vi "Bildaufnahme_Oben.vi"(8 "Fehler in":errorcluster, 11 "Cluster in":T1={"Initialisierung"={"Online?"=FALSE, "Grundpfad"=path "", "Kamera Oben"="", "IP-Adresse Flüssiglinse"="", "Flüssiglinse"=refnum, "Kamera Unten"="", "IP-Adresse SPS"="", "SPS-Verbindung"={"TCP Connection Ref"=refnum, "IP address"="", "timeout ms"=5000, "Connected?"=FALSE, "PLC Type"=enum."S7 1200", "Rack S7 400"=0, "Slot S7 400"=0, "PDU Size"=0, "connection semaphore"=refnum}, "IP-Adresse Lichtgitter"="", "Lichtgitter"=refnum, "Skalierungsfaktor"=0.0, "Bilder Oben"=[], "Bild Unten"=refnum, "Bild Ausschnitt Unten"=refnum}, "Einstellungen"={"Gesamtablauf gestartet"=FALSE, "i. O. Bilder speichern"=FALSE, "Bildspeicherung Offline"=FALSE, "Ausgewähltes Offline-Datum"="", "Ausgewähltes Offline-Teil"="", "Speicherpfad Bilder"=path ""}, "Artikeldaten"={"Artikelnummer"="", "Fertigungsauftrag"="", "Muster ISO"=refnum, "Belichtungszeit Referenzmarken"=0.0, "Fokus Referenzmarken"=0.0, "Belichtungszeit ISO"=0.0, "Fokus ISO"=0.0, "Belichtungszeit Unten"=0.0, "Kontaktanzahl"=0, "Aktueller Kontakt"=0, "Kontaktposition"={"x"=0.0, "y"=0.0}, "Winkel ISO"=0.0, "ISO-Muster nicht vorhanden"=FALSE}, "Werte Kamera Oben"={"Koordinatensystem"={"Punkt x-Achse"={"X"=0.0, "Y"=0.0}, "Ursprung"={"X"=0.0, "Y"=0.0}, "Punkt y-Achse"={"X"=0.0, "Y"=0.0}}, "Position Kontakt"={"x"=0.0, "y"=0.0}, "Winkel Kontakt"=0.0}, "Werte Kamera Unten"={"Prüfung Unten n. i. O."=FALSE}, "Werte Lichtgitter"={"Messwerte Referenzmarken"=[], "Mittelpunkt Referenzmarken"={"x"=0.0, "y"=0.0}, "Messwerte Kontakt"=[], "Offset"={"x"=0.0, "y"=0.0}}, "Rückmeldungen"={"Koordinaten ermittelt"=FALSE, "Vermessung Lichtgitter fertig"=FALSE, "Nachkontrolle Kamera Unten fertig"=FALSE}, "Fehler"={"Referenzen nicht gefunden"=FALSE, "Kontakt nicht gefunden"=FALSE, "Referenzen nicht in Lichtgitter"=FALSE, "Kontakt zu groß"=FALSE, "Kontakt zu klein"=FALSE}, "Statistik"={"Statistiken"=[]}, "Timer"={"Timer Start Position"=0, "Timer Start Lichtgitter"=0, "Timer Start Kamera Unten"=0}}) -> (0 "Fehler out":errorcluster, 3 "Cluster out":T1={"Initialisierung"={"Online?"=FALSE, "Grundpfad"=path "", "Kamera Oben"="", "IP-Adresse Flüssiglinse"="", "Flüssiglinse"=refnum, "Kamera Unten"="", "IP-Adresse SPS"="", "SPS-Verbindung"={"TCP Connection Ref"=refnum, "IP address"="", "timeout ms"=5000, "Connected?"=FALSE, "PLC Type"=enum."S7 1200", "Rack S7 400"=0, "Slot S7 400"=0, "PDU Size"=0, "connection semaphore"=refnum}, "IP-Adresse Lichtgitter"="", "Lichtgitter"=refnum, "Skalierungsfaktor"=0.0, "Bilder Oben"=[], "Bild Unten"=refnum, "Bild Ausschnitt Unten"=refnum}, "Einstellungen"={"Gesamtablauf gestartet"=FALSE, "i. O. Bilder speichern"=FALSE, "Bildspeicherung Offline"=FALSE, "Ausgewähltes Offline-Datum"="", "Ausgewähltes Offline-Teil"="", "Speicherpfad Bilder"=path ""}, "Artikeldaten"={"Artikelnummer"="", "Fertigungsauftrag"="", "Muster ISO"=refnum, "Belichtungszeit Referenzmarken"=0.0, "Fokus Referenzmarken"=0.0, "Belichtungszeit ISO"=0.0, "Fokus ISO"=0.0, "Belichtungszeit Unten"=0.0, "Kontaktanzahl"=0, "Aktueller Kontakt"=0, "Kontaktposition"={"x"=0.0, "y"=0.0}, "Winkel ISO"=0.0, "ISO-Muster nicht vorhanden"=FALSE}, "Werte Kamera Oben"={"Koordinatensystem"={"Punkt x-Achse"={"X"=0.0, "Y"=0.0}, "Ursprung"={"X"=0.0, "Y"=0.0}, "Punkt y-Achse"={"X"=0.0, "Y"=0.0}}, "Position Kontakt"={"x"=0.0, "y"=0.0}, "Winkel Kontakt"=0.0}, "Werte Kamera Unten"={"Prüfung Unten n. i. O."=FALSE}, "Werte Lichtgitter"={"Messwerte Referenzmarken"=[], "Mittelpunkt Referenzmarken"={"x"=0.0, "y"=0.0}, "Messwerte Kontakt"=[], "Offset"={"x"=0.0, "y"=0.0}}, "Rückmeldungen"={"Koordinaten ermittelt"=FALSE, "Vermessung Lichtgitter fertig"=FALSE, "Nachkontrolle Kamera Unten fertig"=FALSE}, "Fehler"={"Referenzen nicht gefunden"=FALSE, "Kontakt nicht gefunden"=FALSE, "Referenzen nicht in Lichtgitter"=FALSE, "Kontakt zu groß"=FALSE, "Kontakt zu klein"=FALSE}, "Statistik"={"Statistiken"=[]}, "Timer"={"Timer Start Position"=0, "Timer Start Lichtgitter"=0, "Timer Start Kamera Unten"=0}})   [LabVIEW 2024]
doc: "Nimmt die Bilder für die Prüfung Oben auf, bzw. lädt die Bilder aus den Dateien wenn im \"Offline-Modus\"."
uses:
  Cluster.ctl
  Kontaktmontagemodul.exe/1abvi3w/vi.lib/userDefined/High Color/IMAQdx.ctl
  Kontaktmontagemodul.exe/1abvi3w/vi.lib/DATA AHEAD/SP7/typedefs/S7 Connection.ctl
  Kontaktmontagemodul.exe/1abvi3w/vi.lib/DATA AHEAD/SP7/typedefs/PLC Type.ctl
  Kontaktmontagemodul.exe/1abvi3w/vi.lib/vision/Image Controls.llb/IMAQ Image.ctl
  Koordinatensystem.ctl
  Statistik.ctl
  Kontaktmontagemodul.exe/1abvi3w/vi.lib/vision/driver/IMAQdx.llb/IMAQdx Buffer Number Mode.ctl
  <resource>/objmgr/imaqdx.rc
  Kontaktmontagemodul.exe/1abvi3w/vi.lib/vision/driver/NI_Vision_Acquisition_Software.lvlib
  Kontaktmontagemodul.exe/1abvi3w/vi.lib/vision/NI_Vision_Development_Module.lvlib
  Kontaktmontagemodul.exe/1abvi3w/vi.lib/DATA AHEAD/SP7/SP7.lvlib
panel:
  in  "Angle":i32
  in  "Angle inkrement":i32
  in  "Zeit für Fokus":u32=300
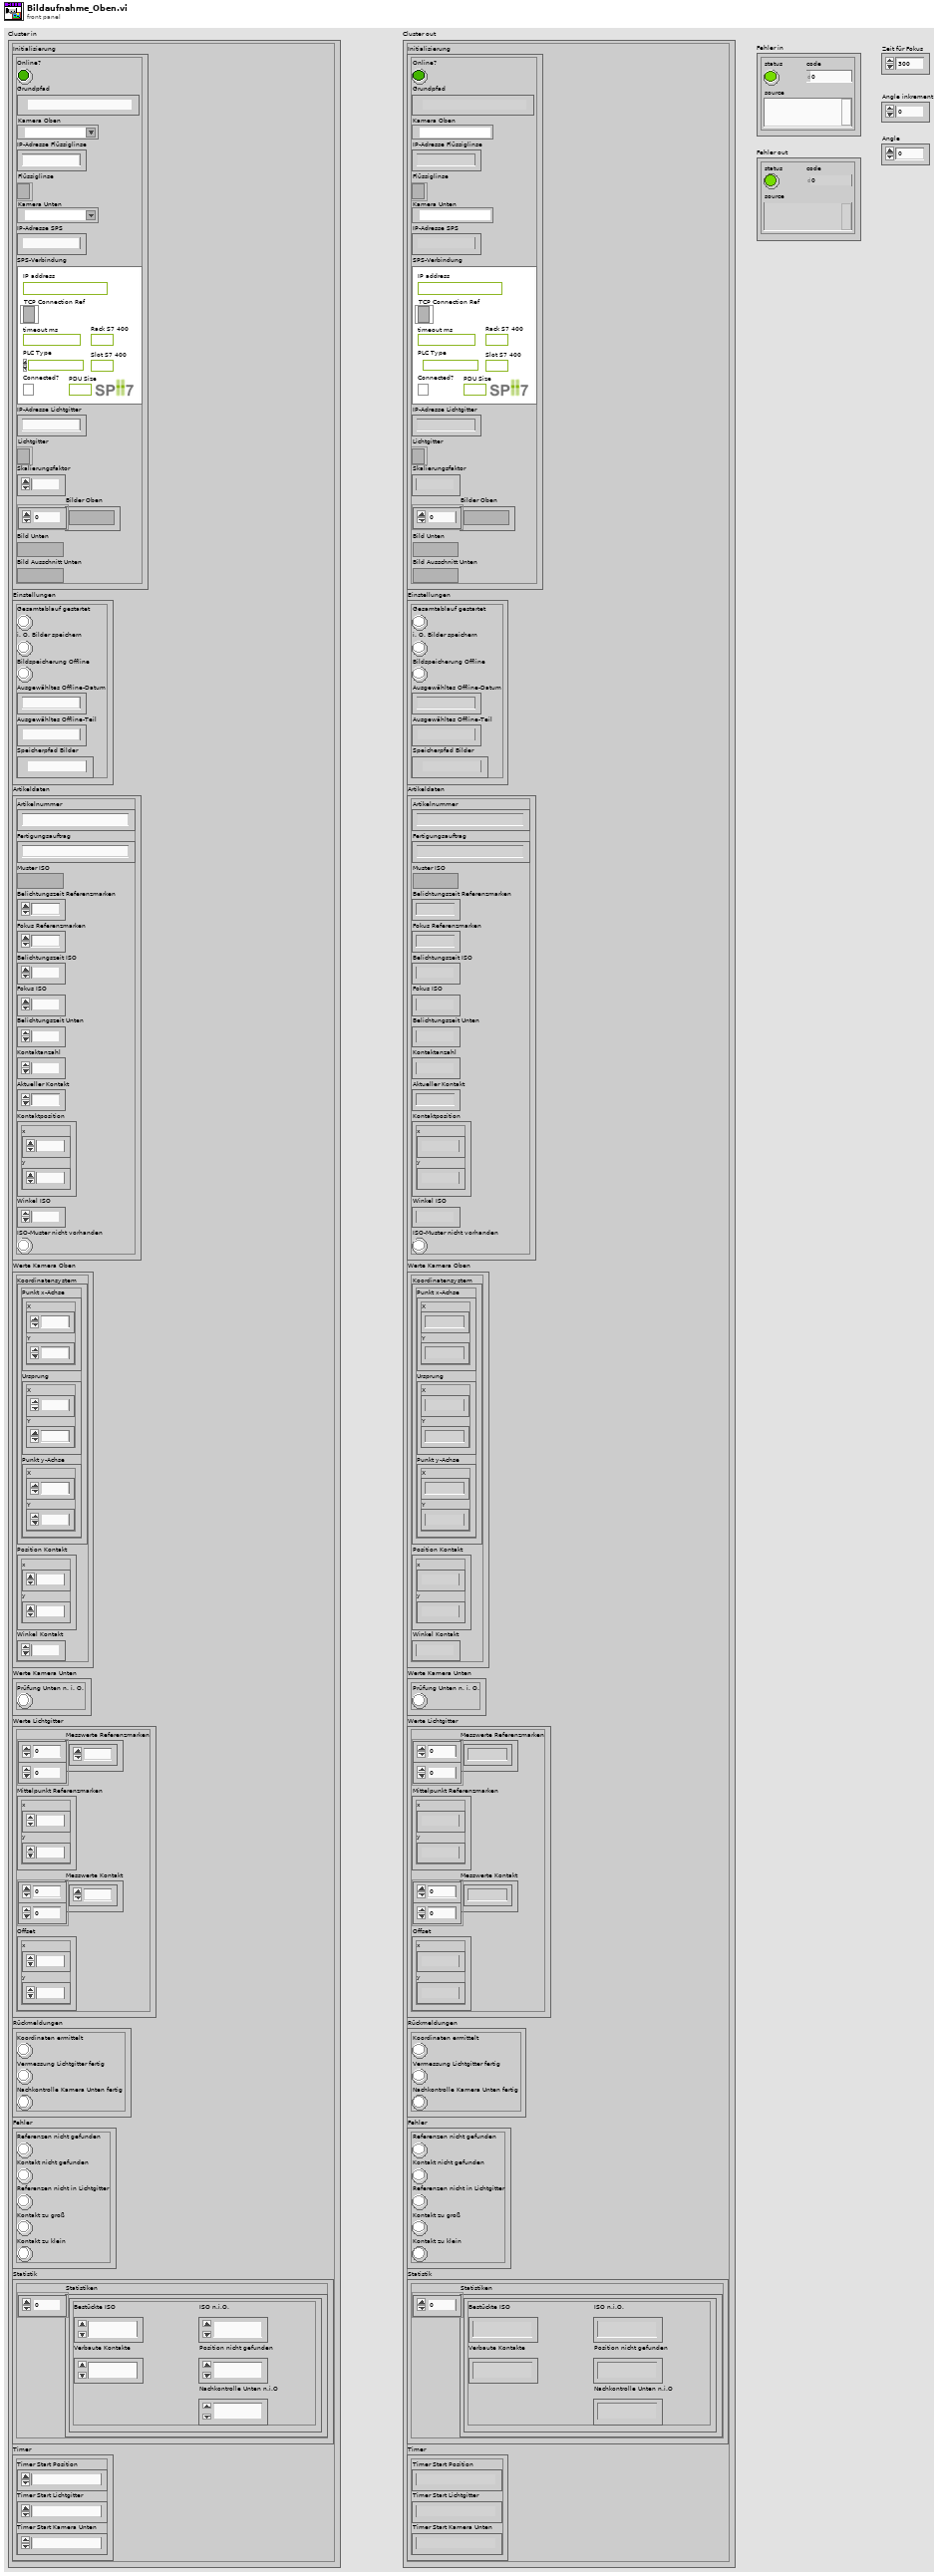
[diagram p1: front panel]
types:
  T1 = typedef "Cluster.ctl" = cluster{"Initialisierung":cluster{"Online?":bool, "Grundpfad":path, "Kamera Oben":T2, "IP-Adresse Flüssiglinse":string, "Flüssiglinse":refnum<k5>, "Kamera Unten":T2, "IP-Adresse SPS":string, "SPS-Verbindung":T3, "IP-Adresse Lichtgitter":string, "Lichtgitter":refnum<k5>, "Skalierungsfaktor":dbl, "Bilder Oben":T6[], "Bild Unten":T6, "Bild Ausschnitt Unten":T6}, "Einstellungen":cluster{"Gesamtablauf gestartet":bool, "i. O. Bilder speichern":bool, "Bildspeicherung Offline":bool, "Ausgewähltes Offline-Datum":string, "Ausgewähltes Offline-Teil":string, "Speicherpfad Bilder":path}, "Artikeldaten":cluster{"Artikelnummer":string, "Fertigungsauftrag":string, "Muster ISO":T6, "Belichtungszeit Referenzmarken":dbl, "Fokus Referenzmarken":dbl, "Belichtungszeit ISO":dbl, "Fokus ISO":dbl, "Belichtungszeit Unten":dbl, "Kontaktanzahl":u32, "Aktueller Kontakt":i16, "Kontaktposition":cluster{"x":sgl, "y":sgl}, "Winkel ISO":sgl, "ISO-Muster nicht vorhanden":bool}, "Werte Kamera Oben":cluster{"Koordinatensystem":T7, "Position Kontakt":cluster{"x":dbl, "y":dbl}, "Winkel Kontakt":dbl}, "Werte Kamera Unten":cluster{"Prüfung Unten n. i. O.":bool}, "Werte Lichtgitter":cluster{"Messwerte Referenzmarken":dbl[][], "Mittelpunkt Referenzmarken":cluster{"x":dbl, "y":dbl}, "Messwerte Kontakt":dbl[][], "Offset":cluster{"x":dbl, "y":dbl}}, "Rückmeldungen":cluster{"Koordinaten ermittelt":bool, "Vermessung Lichtgitter fertig":bool, "Nachkontrolle Kamera Unten fertig":bool}, "Fehler":cluster{"Referenzen nicht gefunden":bool, "Kontakt nicht gefunden":bool, "Referenzen nicht in Lichtgitter":bool, "Kontakt zu groß":bool, "Kontakt zu klein":bool}, "Statistik":cluster{"Statistiken":T8[]}, "Timer":cluster{"Timer Start Position":u32, "Timer Start Lichtgitter":u32, "Timer Start Kamera Unten":u32}}
  T2 = typedef "IMAQdx.ctl" = refnum<k21>
  T3 = typedef "SP7.lvlib/S7 Connection.ctl" = cluster{"TCP Connection Ref":refnum<k5>, "IP address":string, "timeout ms":i32, "Connected?":bool, "PLC Type":T4, "Rack S7 400":u8, "Slot S7 400":u8, "PDU Size":u16, "connection semaphore":T5}
  T4 = typedef "SP7.lvlib/PLC Type.ctl" = enum16{"S7 200", "S7 300/400", "S7 1200", "S7 1500", "LOGO!8"}
  T5 = typedef "Semaphore RefNum" = refnum<k1>
  T6 = typedef "IMAQ Image.ctl" = refnum<image>
  T7 = typedef "Koordinatensystem.ctl" = cluster{"Punkt x-Achse":cluster{"X":sgl, "Y":sgl}, "Ursprung":cluster{"X":sgl, "Y":sgl}, "Punkt y-Achse":cluster{"X":sgl, "Y":sgl}}
  T8 = typedef "Statistik.ctl" = cluster{"Bestückte ISO":u32, "Verbaute Kontakte":u32, "ISO n.i.O.":u32, "Nachkontrolle Unten n.i.O":u32, "Position nicht gefunden":u32}
  T9 = typedef "IMAQ Rectangle" = cluster{"Left":i32, "Top":i32, "Right":i32, "Bottom":i32, "Rotation":dbl}
  T10 = typedef "NI_Vision_Acquisition_Software.lvlib/IMAQdx Buffer Number Mode.ctl" = enum32{"Next", "Last", "Buffer Number", "Every", "Last New"}
  T11 = typedef "ROI Descriptor" = cluster{"Global Rectangle":i32[], "Contours":cluster{"ID":enum32{"External", "Internal"}, "Type":u32, "Coordinates":i32[]}[]}
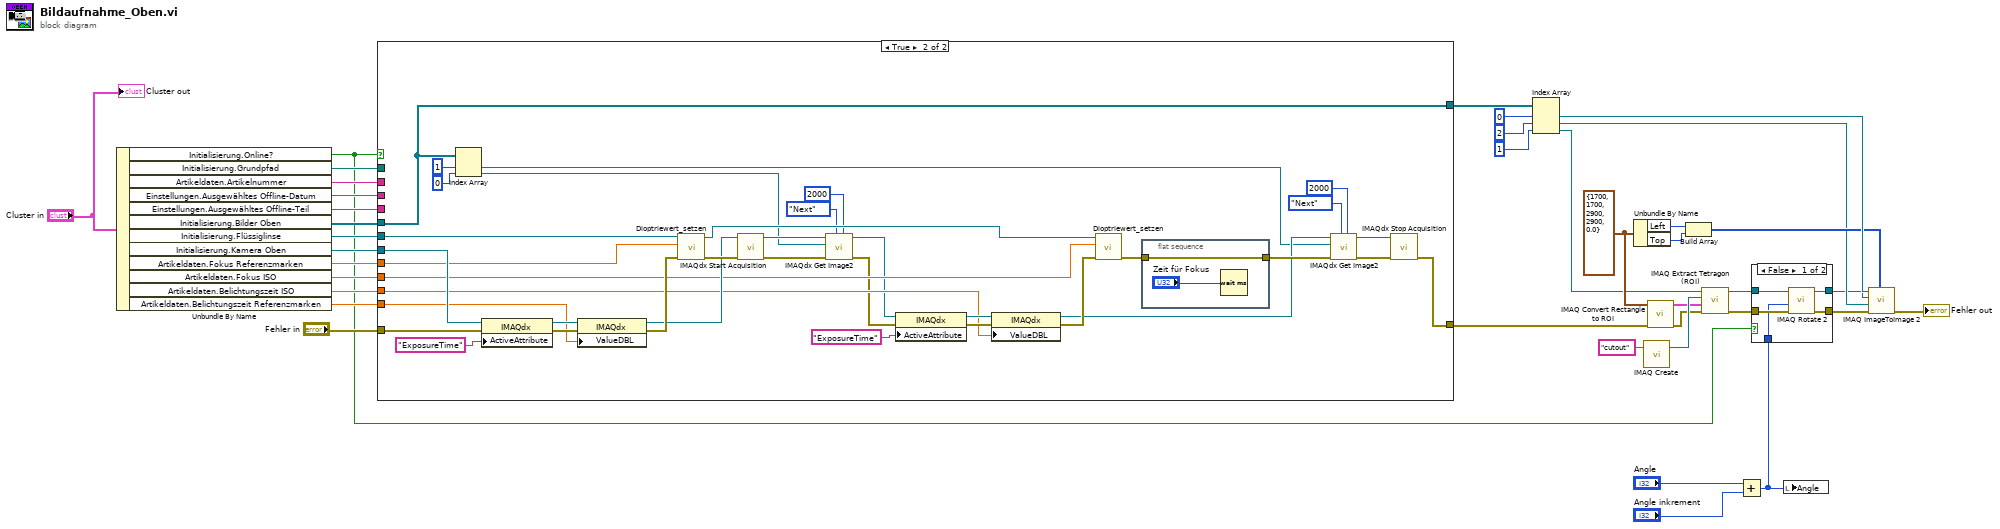
[diagram p0: block diagram]
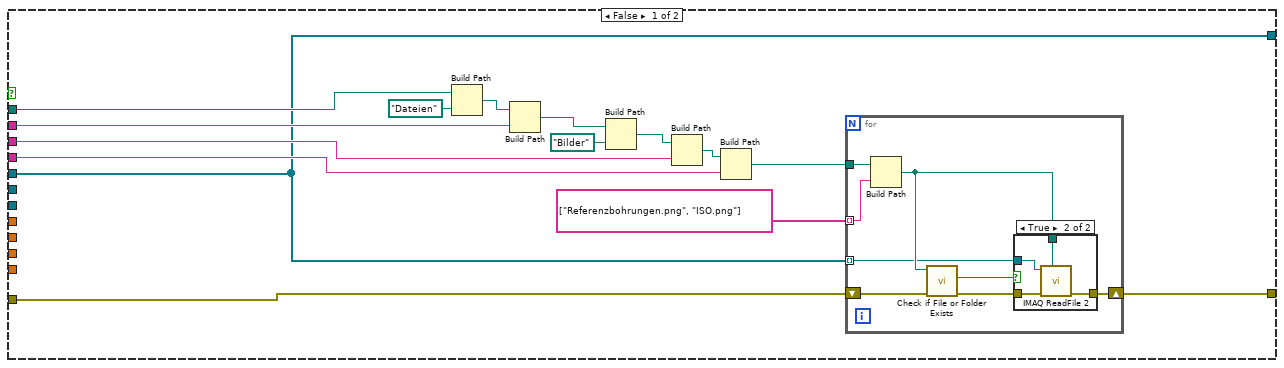
[diagram p3: hidden frame]
diagram:
  w11 = T9 {"Left"=1700, "Top"=1700, "Right"=2900, "Bottom"=2900, "Rotation"=0.0} ("Rectangle")
  n1 = Unbundle By Name("Cluster in") -> ("Initialisierung.Online?"=w1:bool, "Initialisierung.Grundpfad"=w38:path, "Artikeldaten.Artikelnummer"=w37:string, "Einstellungen.Ausgewähltes Offline-Datum"=w35:string, "Einstellungen.Ausgewähltes Offline-Teil"=w36:string, "Initialisierung.Bilder Oben"=w34:T6[], "Initialisierung.Flüssiglinse"=w24:refnum<k5>, "Initialisierung.Kamera Oben"=w23:T2, "Artikeldaten.Fokus Referenzmarken"=w25:dbl, "Artikeldaten.Fokus ISO"=w26:dbl, "Artikeldaten.Belichtungszeit ISO"=w28:dbl, "Artikeldaten.Belichtungszeit Referenzmarken"=w27:dbl)
  n2 = case shown="True" w1 {
    tunnel: w38 -> [w45 _]
    tunnel: w37 -> [w42 _]
    tunnel: w35 -> [w50 _]
    tunnel: w36 -> [w51 _]
    tunnel: w34 -> [w39 w67]
    tunnel: "Fehler in" -> [w47 w87]
    tunnel: [w40 w101] -> w31
    tunnel: [w39 w67] -> w29
    tunnel: w28 -> [_ w80]
    tunnel: w27 -> [_ w81]
    tunnel: w26 -> [_ w79]
    tunnel: w25 -> [_ w84]
    tunnel: w24 -> [_ w86]
    tunnel: w23 -> [_ w85]
    frame False {
      n3 = Build Path(base path=w45, name or relative path=path "Dateien") -> (appended path=w44:path)
      n4 = Build Path(base path=w44, name or relative path=w42) -> (appended path=w53:path)
      n5 = Build Path(base path=w53, name or relative path=path "Bilder") -> (appended path=w46:path)
      n6 = Build Path(base path=w46, name or relative path=w50) -> (appended path=w52:path)
      n7 = Build Path(base path=w52, name or relative path=w51) -> (appended path=w49:path)
      n8 = for {
        tunnel: w39 -> [w55] mode=indexing
        shift-right: [w59] -> w40
        shift-left: w47 -> [w58]
        tunnel: w49 -> [w61]
        tunnel: string[] ["Referenzbohrungen.png", "ISO.png"] -> [w60] mode=indexing
        n9 = Build Path(base path=w61, name or relative path=w60) -> (appended path=w56:path)
        n10 = call "Check if File or Folder Exists.vi"("error in (no error)"=w58, "path"=w56) -> ("error out"=w57:errorcluster, "file or folder exists?"=w54:bool)  [unwired: 7 in, 1 out]
        n11 = case shown="True" w54 {
          tunnel: [w62 w66] -> w59
          tunnel: w57 -> [w62 w65]
          tunnel: w56 -> [_ w64]
          tunnel: w55 -> [_ w63]
          frame False {
          }
          frame True {
            n12 = call "IMAQ ReadFile 2"("File Path"=w64, "error in (no error)"=w65, "Image"=w63) -> ("error out"=w66:errorcluster)  [unwired: 4 in, 4 out]
          }
        }
      }
    }
    frame True {
      n13 = Index Array(array=w67, index #1=1 ("index"), index #2=0 ("index")) -> (element #1=w68:T6, element #2=w69:T6)
      n14 = property class="IMAQdx"(reference=w85, error in=w87, "ActiveAttribute"="ExposureTime") -> (reference out=w90:T2, error out=w89:errorcluster)
      n15 = property class="IMAQdx"(reference=w90, error in=w89, "ValueDBL"=w81) -> (reference out=w83:T2, error out=w91:errorcluster)
      n16 = call "Dioptriewert_setzen.vi"("Fehler in"=w91, "Dioptrie-Wert"=w84, "Flüssiglinse in"=w86) -> ("Fehler out"=w88:errorcluster, "Flüssiglinse out"=w78:refnum<k5>)  [unwired: 7 in]
      n17 = call "IMAQdx Start Acquisition.vi"("error in"=w88, "Session In"=w83) -> ("error out"=w75:errorcluster, "Session Out"=w73:T2)  [unwired: 8 in]
      n18 = call "IMAQdx Get Image2.vi"("Timeout (ms)"=2000, "Buffer Number Mode (Next)"=IMAQdx_Buffer_Number_Mode."Next", "error in"=w75, "Image In"=w69, "Session In"=w73) -> ("error out"=w74:errorcluster, "Session Out"=w72:T2)  [unwired: 3 in, 2 out]
      n19 = property class="IMAQdx"(reference=w72, error in=w74, "ActiveAttribute"="ExposureTime") -> (reference out=w99:T2, error out=w100:errorcluster)
      n20 = property class="IMAQdx"(reference=w99, error in=w100, "ValueDBL"=w80) -> (reference out=w94:T2, error out=w97:errorcluster)
      n21 = call "Dioptriewert_setzen.vi"("Fehler in"=w97, "Dioptrie-Wert"=w79, "Flüssiglinse in"=w78) -> ("Fehler out"=w96:errorcluster)  [unwired: 7 in, 1 out]
      n22 = flat-sequence {
        tunnel: w96 -> [w105]
        tunnel: [w105] -> w95
        frame #0 {
          n23 = Wait (ms)(milliseconds to wait="Zeit für Fokus") -> ()  [unwired: 1 out]
        }
      }
      n24 = call "IMAQdx Get Image2.vi"("Timeout (ms)"=2000, "Buffer Number Mode (Next)"=IMAQdx_Buffer_Number_Mode."Next", "error in"=w95, "Image In"=w68, "Session In"=w94) -> ("error out"=w103:errorcluster, "Session Out"=w102:T2)  [unwired: 3 in, 2 out]
      n25 = call "IMAQdx Stop Acquisition.vi"("error in"=w103, "Session In"=w102) -> ("error out"=w101:errorcluster)  [unwired: 8 in, 1 out]
    }
  }
  n26 = Index Array(array=w29, index #1=0 ("index"), index #2=2 ("index"), index #3=1 ("index")) -> (element #1=w21:T6, element #2=w10:T6, element #3=w9:T6)
  n27 = Unbundle By Name(w11) -> ("Left"=w18:i32, "Top"=w17:i32)
  n28 = call "IMAQ Create"("Image Name"="cutout") -> ("New Image"=w22:T6)  [unwired: 4 in, 1 out]
  n29 = call "IMAQ Convert Rectangle to ROI"("error in (no error)"=w31, "Rectangle"=w11) -> ("error out"=w19:errorcluster, "ROI Descriptor"=w20:T11)  [unwired: 7 in]
  n30 = Build Array(w18, w17) -> (w16:i32[])
  n31 = call "IMAQ Extract Tetragon (ROI)"("error in (no error)"=w19, "ROI Descriptor"=w20, "Image Dst"=w22, "Image Src"=w9) -> ("error out"=w7:errorcluster, "Image Dst Out"=w8:T6)  [unwired: 6 in]
  n32 = Add(x="Angle", y="Angle inkrement") -> (x+y=w2:i32)
  n33 = case shown="False" w1 {
    tunnel: w8 -> [w110 w112]
    tunnel: w7 -> [w109 w111]
    tunnel: [w108 w112] -> w6
    tunnel: [w107 w111] -> w5
    tunnel: w2 -> [w106 _]
    frame False {
      n34 = call "IMAQ Rotate 2"("error in (no error)"=w109, "Angle (degrees)"=w106, "Image Src"=w110) -> ("error out"=w107:errorcluster, "Image Dst Out"=w108:T6)  [unwired: 7 in]
    }
    frame True {
    }
  }
  n35 = local write "Angle"(w2) -> ()
  n36 = call "IMAQ ImageToImage 2"("Offset Left/Top"=w16, "error in (no error)"=w5, "Image Dst"=w10, "Image Src (Small)"=w6, "Image Src (Large)"=w21) -> ("error out"=→"Fehler out":errorcluster)  [unwired: 5 in, 1 out]
  "Cluster out" <- "Cluster in"
